vi "Configure Integration Real Time.vi"(0 "VISA resource name":refnum<visa-resource-name>, 2 "Start/End (0: Start)":i32(ring) items=["Start", "End"], 3 "Element (0: ALL)":i32(ring) items=["All", "1", "2", "3", "4", "5", "6"], 11 "error in (no error)":errorcluster) -> (4 "VISA resource name out":refnum<visa-resource-name>, 15 "error out":errorcluster)   [LabVIEW 2021, in "Yokogawa WT1800 Series.lvlib"]
doc: "Configures the integration real-time features.\n\n<b>Note:</b>\nThis setting valid when the <b>Integration Mode</b> in the <b>Configure Integration</b> VI is <b>Real-time Normal</b> or <b>Real-time Continuous</b>."
uses:
  <instrlib>/Yokogawa WT1800 Series/Yokogawa WT1800 Series.lvlib
panel:
  in  "Time Stamp (00:00:00:2001/01/01)":timestamp=timestamp(3061119600.078 s since 1904-01-01) format="%<%X\n%x>T"
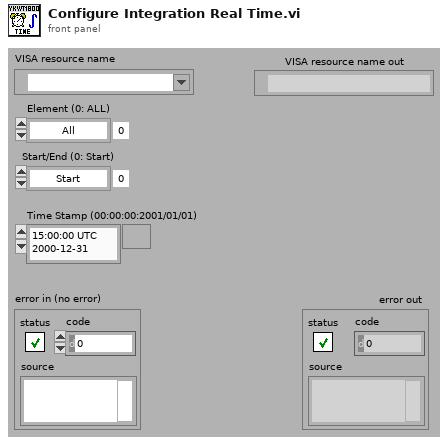
[diagram p1: front panel]
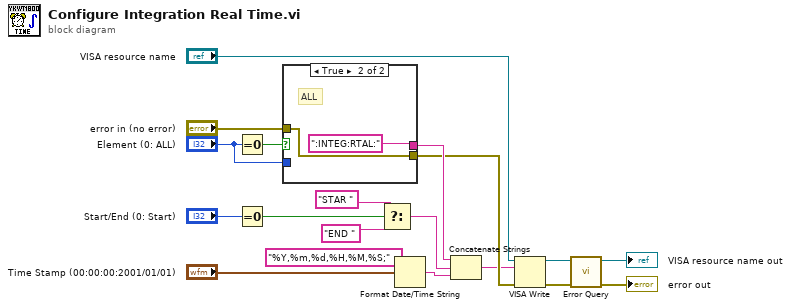
[diagram p0: block diagram]
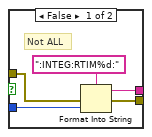
[diagram p2: hidden frame]
diagram:
  n1 = Equal To 0?(x="Element (0: ALL)") -> (x = 0?=w14:bool)
  n2 = Equal To 0?(x="Start/End (0: Start)") -> (x = 0?=w8:bool)
  n3 = case shown="True" w14 {
    tunnel: "error in (no error)" -> [w23 w26]
    tunnel: [w22 w26] -> w3
    tunnel: [w21 ":INTEG:RTAL:"] -> w6
    tunnel: "Element (0: ALL)" -> [w20 _]
    frame False {
      # "Not ALL"
      n4 = Format Into String ("文字列にフォーマット")(format string=":INTEG:RTIM%d:" ("形式文字列"), error in=w23, w20) -> (resulting string=w21:string, error out=w22:errorcluster)  [unwired: 1 in]
    }
    frame True {
      # "ALL"
    }
  }
  n5 = Select(t="STAR ", s=w8, f="END ") -> (s? t:f=w7:string)
  n6 = Format Date/Time String(time format string (%c)="%Y,%m,%d,%H,%M,%S;" ("Ô`®¶ñi%cj"), seconds (now)="Time Stamp (00:00:00:2001/01/01)") -> (date/time string=w2:string)  [unwired: 1 in]
  n7 = Concatenate Strings(w6, w7, w2) -> (w1:string)
  n8 = VISA Write ("VISA書き込み")(VISA resource name="VISA resource name", write buffer=w1, error in (no error)=w3) -> (VISA resource name out=w19:refnum<visa-resource-name>, error out=w18:errorcluster)  [unwired: 1 out]
  n9 = call <instrlib>:"Error Query.vi"("error in (no error)"=w18, "VISA resource name"=w19) -> ("error out"=→"error out":errorcluster, "VISA resource name out"=→"VISA resource name out":refnum<visa-resource-name>)  [unwired: 6 in, 2 out]
